vi "Read Enabled Values.vi"(8 "error in (no error)":errorcluster, 11 "No Out in":refnum<class "No Output.lvclass">) -> (0 "error out":errorcluster, 1 "Data Values Native":dbl[](array[numeric]), 2 "Data Values Engineering":dbl[](array[numeric]), 3 "No Out out":refnum<class "No Output.lvclass">)   [LabVIEW 2018, in "No Output.lvclass"]
uses:
  No Output.lvclass
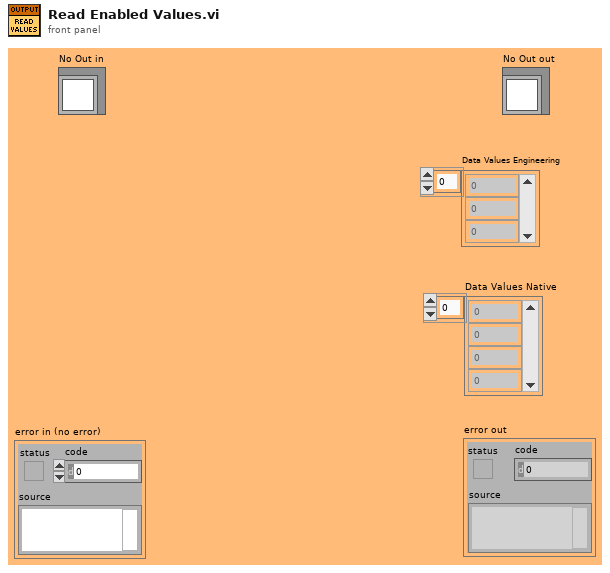
[diagram p1: front panel]
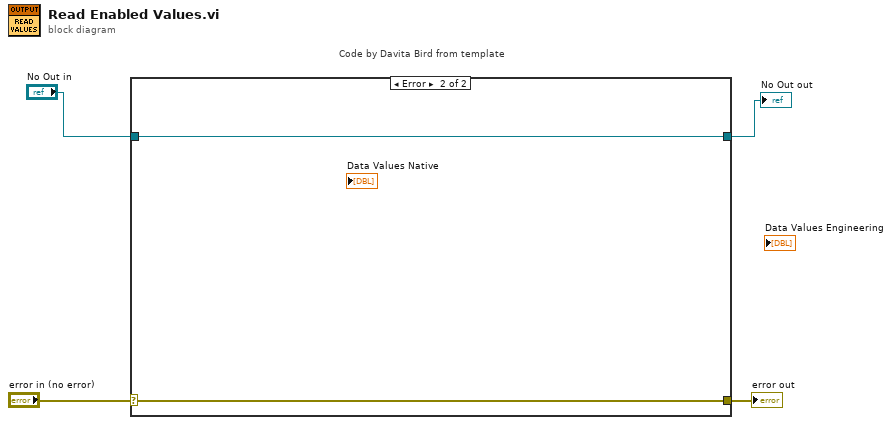
[diagram p0: block diagram]
diagram:
  n1 = case "Code by Davita Bird from template" shown="Error" "error in (no error)" {
    selector: "error in (no error)" -> [w5 w8]
    tunnel: [w5 w8] -> w3
    tunnel: [w6 w7] -> w2
    tunnel: "No Out in" -> [w6 w7]
    frame No Error {
    }
    frame Error {
    }
  }
  "error out" <- w3
  "No Out out" <- w2
